vi "Result_Test.vi"(8 "error in (no error)":errorcluster caption="entrée d'erreur (pas d'erreur)", 11 "Flash_Jlink en entrée":refnum<class "P2265_Boot_IEEE.lvclass">) -> (0 "error out":errorcluster caption="sortie d'erreur", 3 "Flash_Jlink en sortie":refnum<class "P2265_Boot_IEEE.lvclass">)   [LabVIEW 2020, in "Library Test.lvlib" / "P2265_Boot_IEEE.lvclass"]
uses:
  P2265_Boot_IEEE.lvclass
  C:/Users/ngarcin/OneDrive - Altyor/Standard TB/Class/Test/Test (Default)/Test (Default).lvclass
  JSON API/JSON Value/Set from JSON string.vi
  JSON API/JSON Value/JSON Value.lvclass
  Test_Without_Instr/Test_Without_Inst.lvclass
  P2265_Boot_IEEE.lvclass/P2265_Boot_IEEE.ctl
  JSON API/Variant JSON/Variant JSON.lvlib
  JSON API/Get Polymorphic/JSON GetSet.lvlib
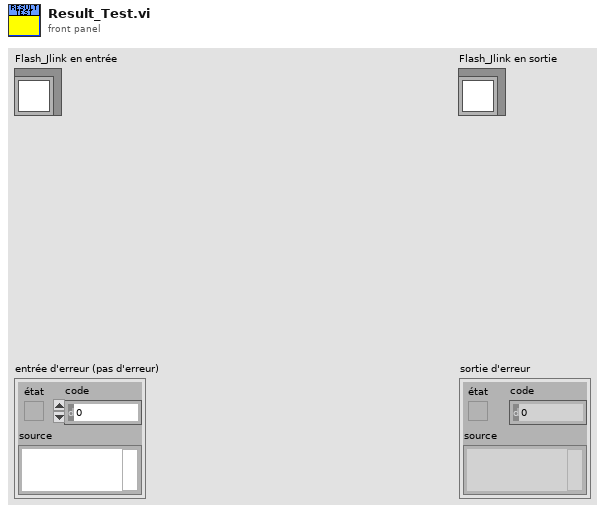
[diagram p1: front panel]
types:
  T1 = cluster{"FW Version":string, "IEE Address":string}
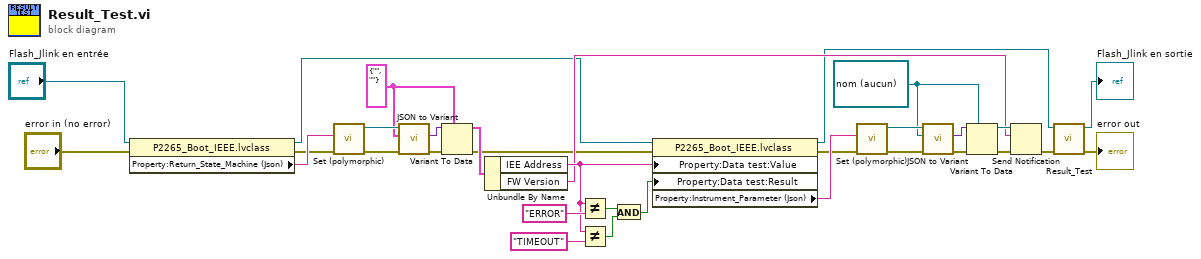
[diagram p0: block diagram]
diagram:
  w9 = T1 {"FW Version"="", "IEE Address"=""} ("Cluster des données privées de classe")
  w19 = refnum<notifier> refnum ("notificateur en sortie")
  n1 = property class="P2265_Boot_IEEE.lvclass"(reference="Flash_Jlink en entrée", error in="error in (no error)") -> (reference out=w4:refnum<class "P2265_Boot_IEEE.lvclass">, error out=w3:errorcluster, "Property:Return_State_Machine (Json)"=w7:string)
  n2 = call-poly "Set (polymorphic).vi"("error in (no error)"=w3, "JSON stream"=w7) -> ("error out"=w11:errorcluster, "JSON Value out"=w13:refnum<class "JSON Value.lvclass">)  [unwired: 7 in, 1 out]
  n3 = call "JSON to Variant.vi"("error in (no error)"=w11, "Variant (Data Type)"=w9, "JSON Value"=w13) -> ("error out"=w12:errorcluster, "Variant out"=w10:variant)  [unwired: 7 in]
  n4 = Variant To Data(error in=w12, type=w9, Variant=w10) -> (data=w8:T1, error out=w2:errorcluster)
  n5 = Unbundle By Name(w8) -> ("IEE Address"=w29:string, "FW Version"=w16:string)
  n6 = Not Equal?(x=w29, y="ERROR" ("expression régulière")) -> (x != y?=w28:bool)
  n7 = Not Equal?(x=w29, y="TIMEOUT" ("expression régulière")) -> (x != y?=w27:bool)
  n8 = And(x=w28, y=w27) -> (x .and. y?=w26:bool)
  n9 = property class="P2265_Boot_IEEE.lvclass"(reference=w4, error in=w2, "Property:Data test:Value"=w29, "Property:Data test:Result"=w26) -> (reference out=w1:refnum<class "P2265_Boot_IEEE.lvclass">, error out=w20:errorcluster, "Property:Instrument_Parameter (Json)"=w21:string)
  n10 = call-poly "Set (polymorphic).vi"("error in (no error)"=w20, "JSON stream"=w21) -> ("error out"=w23:errorcluster, "JSON Value out"=w25:refnum<class "JSON Value.lvclass">)  [unwired: 7 in, 1 out]
  n11 = call "JSON to Variant.vi"("error in (no error)"=w23, "Variant (Data Type)"=w19, "JSON Value"=w25) -> ("error out"=w24:errorcluster, "Variant out"=w22:variant)  [unwired: 7 in]
  n12 = Variant To Data(error in=w24, type=w19, Variant=w22) -> (data=w17:refnum<notifier>, error out=w18:errorcluster)
  n13 = Send Notification(notification=w16, notifier=w17, error in (no error)=w18) -> (error out=w14:errorcluster)  [unwired: 1 out]
  n14 = call-parent "Result_Test.vi"("error in (no error)"=w14, "Test_Without_Inst en entrée"=w1) -> ("error out"=→"error out":errorcluster, "Test_Without_Inst en sortie"=→"Flash_Jlink en sortie":refnum<class "P2265_Boot_IEEE.lvclass">)  [unwired: 8 in]
